vi "functions.vi"() -> ()   [LabVIEW 2013]
panel:
  in  "types":string[](array[string])=["double", "float", "int64", "int32", "int16", "int8", "uInt64", "uInt32", "uInt16", "uInt8", "LVBoolean", "LStrHandle"]
  out "lvDataCluster.h":string
  in  "names":string[](array[string])=["Double", "Single", "I64", "I32", "I16", "I8", "U64", "U32", "U16", "U8", "Boolean", "String"]
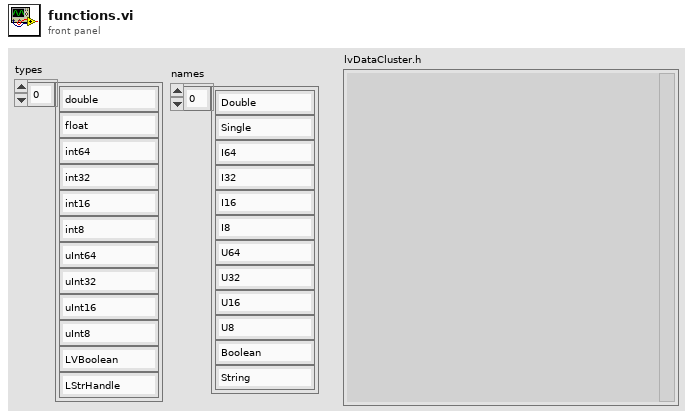
[diagram p1: front panel]
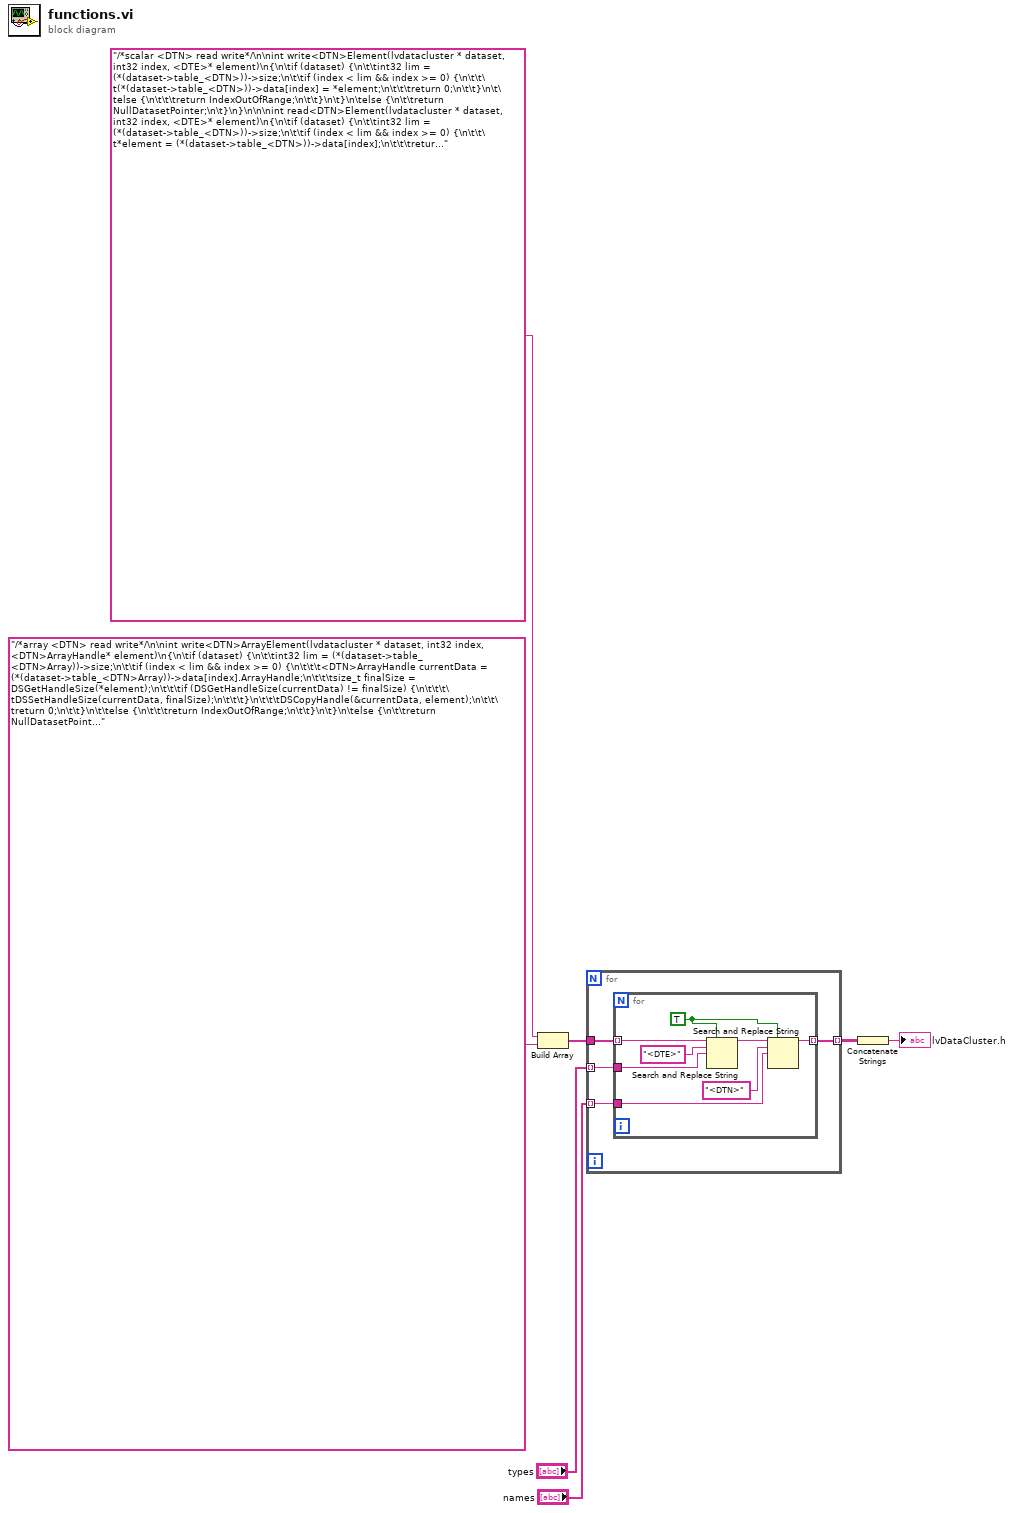
[diagram p0: block diagram]
diagram:
  n1 = Build Array("/*scalar <DTN> read write*/\n\nint write<DTN>Element(lvdatacluster * dataset, int32 index, <DTE>* element)\n{\n\tif (dataset) {\n\t\tint32 lim = (*(dataset->table_<DTN>))->size;\n\t\tif (index < lim && index >= 0) {\n\t\t\t(*(dataset->table_<DTN>))->data[index] = *element;\n\t\t\treturn 0;\n\t\t}\n\t\telse {\n\t\t\treturn IndexOutOfRange;\n\t\t}\n\t}\n\telse {\n\t\treturn NullDatasetPointer;\n\t}\n}\n\n\nint read<DTN>Element(lvdatacluster * dataset, int32 index, <DTE>* element)\n{\n\tif (dataset) {\n\t\tint32 lim = (*(dataset->table_<DTN>))->size;\n\t\tif (index < lim && index >= 0) {\n\t\t\t*element = (*(dataset->table_<DTN>))->data[index];\n\t\t\treturn 0;\n\t\t}\n\t\telse {\n\t\t\treturn IndexOutOfRange;\n\t\t}\n\t}\n\telse {\n\t\treturn NullDatasetPointer;\n\t}\n}\n\n", "/*array <DTN> read write*/\n\nint write<DTN>ArrayElement(lvdatacluster * dataset, int32 index, <DTN>ArrayHandle* element)\n{\n\tif (dataset) {\n\t\tint32 lim = (*(dataset->table_<DTN>Array))->size;\n\t\tif (index < lim && index >= 0) {\n\t\t\t<DTN>ArrayHandle currentData = (*(dataset->table_<DTN>Array))->data[index].ArrayHandle;\n\t\t\tsize_t finalSize = DSGetHandleSize(*element);\n\t\t\tif (DSGetHandleSize(currentData) != finalSize) {\n\t\t\t\tDSSetHandleSize(currentData, finalSize);\n\t\t\t}\n\t\t\tDSCopyHandle(&currentData, element);\n\t\t\treturn 0;\n\t\t}\n\t\telse {\n\t\t\treturn IndexOutOfRange;\n\t\t}\n\t}\n\telse {\n\t\treturn NullDatasetPointer;\n\t}\n}\n\n\nint read<DTN>ArrayElement(lvdatacluster * dataset, int32 index, <DTN>ArrayHandle* element)\n{\n\tif (dataset) {\n\t\tint32 lim = (*(dataset->table_<DTN>Array))->size;\n\t\tif (index < lim && index >= 0) {\n\t\t\t<DTN>ArrayHandle currentData= (*(dataset->table_<DTN>Array))->data[index].ArrayHandle;\n\t\t\tsize_t finalSize = DSGetHandleSize(currentData);\n\t\t\tif (!element) {\n\t\t\t\t<DTN>ArrayHandle t = (<DTN>ArrayHandle) DSNewHandle(finalSize);\n\t\t\t\telement = &t;\n\t\t\t}\n\t\t\telse if (DSGetHandleSize(element) != finalSize) {\n\t\t\t\tDSSetHandleSize(*element, finalSize);\n\t\t\t}\n\t\t\telse {\n\t\t\t}\n\t\t\tDSCopyHandle(element, &currentData);\t\t\t\n\t\t\treturn 0;\n\t\t}\n\t\telse {\n\t\t\treturn IndexOutOfRange;\n\t\t}\n\t}\n\telse {\n\t\treturn NullDatasetPointer;\n\t}\n}\n\n") -> (w2:string[])
  n2 = for {
    tunnel: "types" -> [w11] mode=indexing
    tunnel: "names" -> [w10] mode=indexing
    tunnel: w2 -> [w9]
    tunnel: [w8] -> w6 mode=indexing
    n3 = for {
      tunnel: w11 -> [w13]
      tunnel: w10 -> [w15]
      tunnel: w9 -> [w19] mode=indexing
      tunnel: [w17] -> w8 mode=indexing
      w12 = TRUE ("replace all? (F)")
      n4 = Search and Replace String(replace all?=w12, input string=w19, search string="<DTE>", replace string=w13) -> (result string=w18:string)  [unwired: 4 in, 3 out]
      n5 = Search and Replace String(replace all?=w12, input string=w18, search string="<DTN>", replace string=w15) -> (result string=w17:string)  [unwired: 4 in, 3 out]
    }
  }
  n6 = Concatenate Strings(w6) -> (→"lvDataCluster.h":string)
